vi "TimebaseCfg.vi"(8 "error in (no error)":errorcluster, 10 "Horizontal Settings":T2={"Time/div"=0.01, "Trigger Holdoff"=0.0} {"Time/div" scale=0.0001..1.0 scale format="%#_8g"}, 11 "reference in":refnum<k24>) -> (0 "error out":errorcluster, 1 "[Meta]SetupInfoTrigger":T1, 3 "reference out":refnum<k24>)   [LabVIEW 2019, in "LabNation Scope Driver.lvlib"]
doc: "Set up the Timebase.\nThe Time/div value is in ms."
uses:
  LabNation Scope Driver.lvlib
  C:/Program Files (x86)/LabNation/SmartScope/DeviceInterface.dll
  Program Files (x86)/LabNation/SmartScope/DeviceInterface.dll
  Typedef/Horizontal Settings.ctl
  Typedef/TimeSetting.ctl
  Typedef/Metadata/[Meta]SetupInfoTrigger.ctl
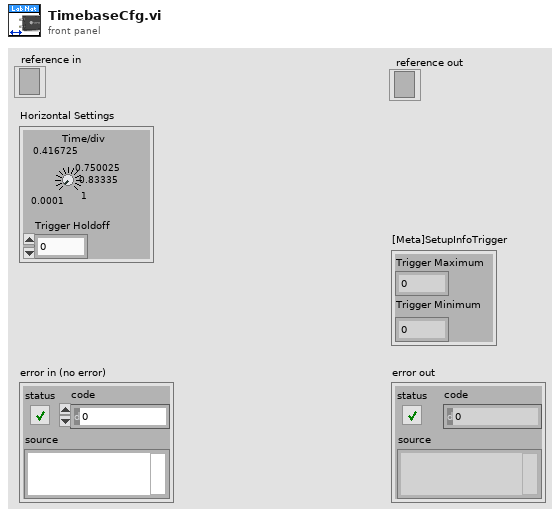
[diagram p1: front panel]
types:
  T1 = typedef "LabNation Scope Driver.lvlib/[Meta]SetupInfoTrigger.ctl" = cluster{"Trigger Maximum":dbl, "Trigger Minimum":dbl}
  T2 = typedef "LabNation Scope Driver.lvlib/Horizontal Settings.ctl" = cluster{"Time/div":T3, "Trigger Holdoff":dbl}
  T3 = typedef "LabNation Scope Driver.lvlib/TimeSetting.ctl" = dbl
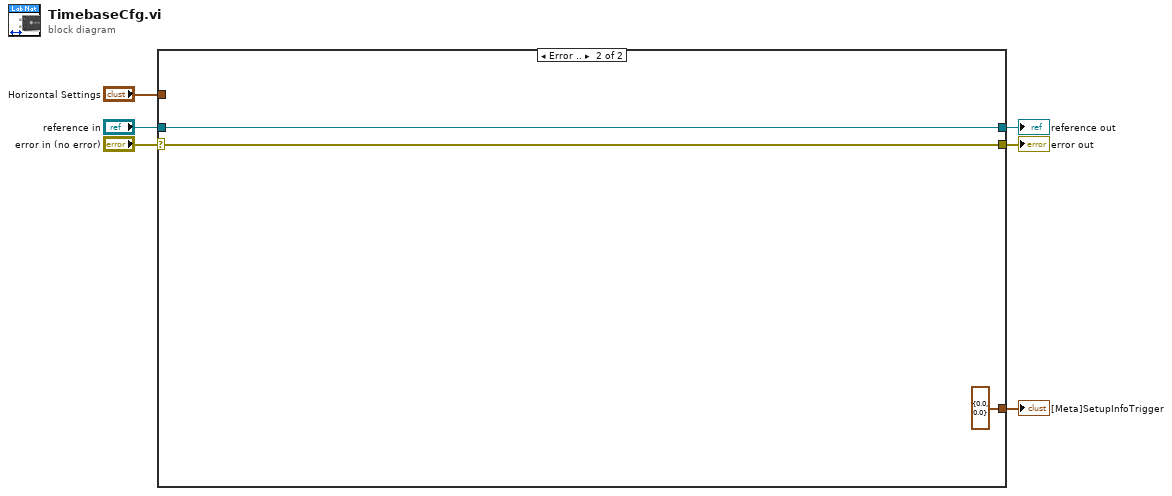
[diagram p0: block diagram]
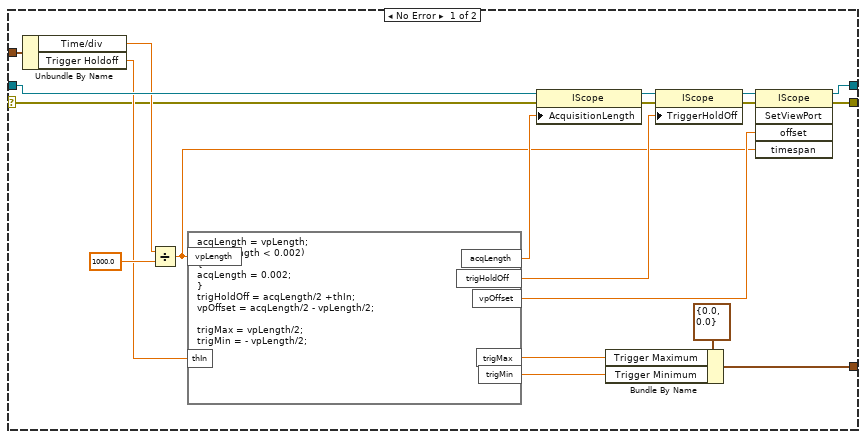
[diagram p2: hidden frame]
diagram:
  n1 = case shown="Error .." "error in (no error)" {
    selector: "error in (no error)" -> [w7 w28]
    tunnel: "reference in" -> [w20 w29]
    tunnel: [w19 w29] -> w5
    tunnel: [w18 w28] -> w4
    tunnel: "Horizontal Settings" -> [w17 _]
    tunnel: [w10 T1 {"Trigger Maximum"=0.0, "Trigger Minimum"=0.0} ("Setup Info Horizontal")] -> w2
    frame No Error {
      n2 = Unbundle By Name(w17) -> ("Time/div"=w16:T3, "Trigger Holdoff"=w14:dbl)
      n3 = Divide(x=w16, y=1000.0) -> (x/y=w15:T3)
      n4 = formula code="acqLength = vpLength;\nif (acqLength < 0.002)\n{\nacqLength = 0.002;\n}\ntrigHoldOff = acqLength/2 +thIn;\nvpOffset = acqLength/2 - vpLength/2;\n\ntrigMax = vpLength/2;\ntrigMin = - vpLength/2;"("vpLength"=w15, "thIn"=w14) -> ("acqLength"=w23:dbl, "trigHoldOff"=w21:dbl, "vpOffset"=w24:dbl, "trigMax"=w9:dbl, "trigMin"=w8:dbl)
      n5 = property class="IScope"(reference=w20, error in=w7, "AcquisitionLength"=w23) -> (reference out=w22:refnum<k24>, error out=w13:errorcluster)
      n6 = Bundle By Name(cluster=T1 {"Trigger Maximum"=0.0, "Trigger Minimum"=0.0} ("Setup Info Horizontal"), "Trigger Maximum"=w9, "Trigger Minimum"=w8) -> (w10:T1)
      n7 = property class="IScope"(reference=w22, error in=w13, "TriggerHoldOff"=w21) -> (reference out=w25:refnum<k24>, error out=w12:errorcluster)
      n8 = invoke class="IScope" method="SetViewPort"(reference=w25, error in=w12, "offset"=w24, "timespan"=w15) -> (reference out=w19:refnum<k24>, error out=w18:errorcluster)  [unwired: 1 in, 3 out]
    }
    frame Error {
    }
  }
  "error out" <- w4
  "reference out" <- w5
  "[Meta]SetupInfoTrigger" <- w2
